vi "BotStatus.vi"() -> ()   [LabVIEW 2012]
panel:
  in  "Ready to Fire":bool
  in  "Calculated zAvit":dbl
  in  "Axis X":dbl
  in  "Whole robot centering":bool
  in  "center on target":bool
  in  "View ground":bool
  in  "Stop auto camera movment":bool
  in  "axis 3 camera controller joystick":dbl
  in  "Y axis camera controller joystick":dbl
  in  "Canenet Right":dbl
  in  "Camera Servo Y":dbl
  in  "Camera Servo X":dbl
  in  "Feeder":dbl
  in  "Canenet Left":dbl
  in  "zAvit":dbl
  in  "Cannon":dbl
  in  "Transfer":dbl
  in  "Conveyer Belt":dbl
  in  "Cannon LS":T1
  in  "Frisbee in Stack Counter":i32
  in  "Target Info":T2
  in  "Frisbee States":T3
  # "Number (0<=X<=3)"
  # "Cannon"
  # "InCannon"
  # "InFlipper"
  # "FlipperAtPlace"
  # "Middle"
  # "Bottom"
  # "UPDATES VALUES IN Periodic Tasks.vi"
  # "Feeder Angle"
  # "Flipper Angle"
  # "Cannon Angle"
  # "90"
  # "90"
  # "90"
  # "131"
  # "170"
  # "170"
  # "0"
  # "48.6 => 49"
  # "0"
  # "-min angle"
  # "0"
  # "\"Cannon Position(deg)\""
  # "(cannon motors)"
  # "VBus"
  # "VBus"
  # "Joystick Axis value"
  # "Irrelevant"
  # "Joystick Axis value"
  # "VBus"
  # "VBus"
  # "VBus"
  # "Joystick Axis value"
  # "Angle"
  # "Relay"
  # "Angle"
  # "Angle"
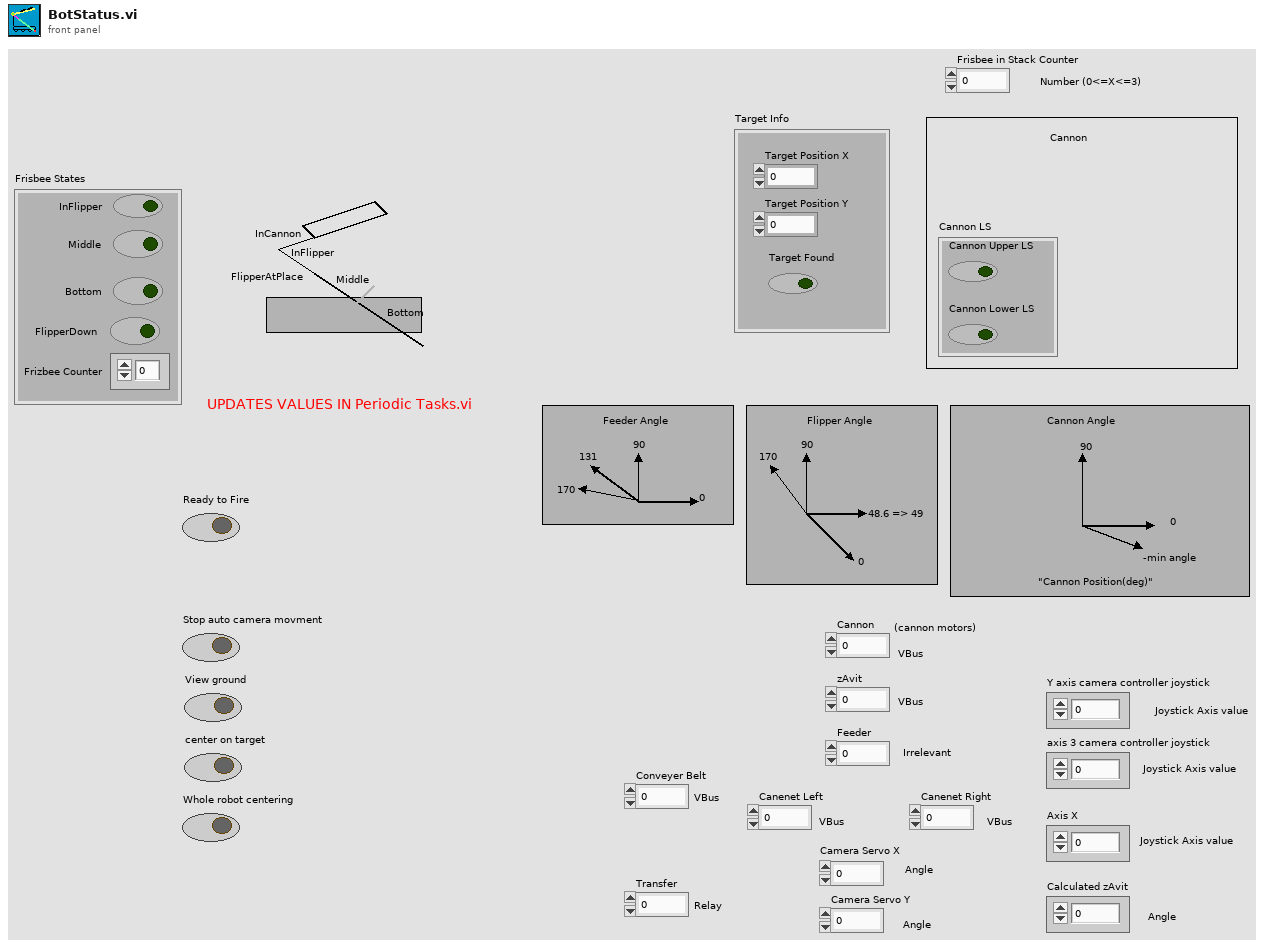
[diagram p1: front panel]
types:
  T1 = cluster{"Cannon Upper LS":bool, "Cannon Lower LS":bool}
  T2 = cluster{"Target Position X":dbl, "Target Position Y":dbl, "Target Found":bool}
  T3 = cluster{"Middle":bool, "InFlipper":bool, "Bottom":bool, "FlipperDown":bool, "Frizbee Counter":dbl}
diagram:
